vi "Init Runtime.vi"(8 "error in (no error)":errorcluster, 10 "data allocations":T1, 11 "Counter Config in":refnum<class "Counter Config.lvclass">) -> (0 "error out":errorcluster, 2 "Skip":bool, 3 "Counter Config out":refnum<class "Counter Config.lvclass">)   [LabVIEW 2015, in "Counter Config.lvclass"]
uses:
  Counter Config.lvclass
  <vilib>/NI/Tag Bus Module Framework/channel/data tables.ctl
  <vilib>/NI/Tag Bus/dictionary/data dictionary.lvclass
  <vilib>/NI/Tag Bus/dictionary table pair.ctl
  <vilib>/NI/Tag Bus/table/data table.ctl
  Runtime/Counter.lvclass
  <vilib>/NI/Tag Bus/tag/tag descriptor.lvclass/tag descriptor.ctl
  <vilib>/NI/Tag Bus/tag/read tag name.vi
  <vilib>/NI/Tag Bus/tag/read data type.vi
  <vilib>/NI/Tag Bus/dictionary/locate tag.vi
  <vilib>/NI/Tag Bus Module Framework/channel/TBM channel.lvclass
  <vilib>/NI/Tag Bus/table/data table.lvlib
  <vilib>/NI/Tag Bus/tag bus.lvlib
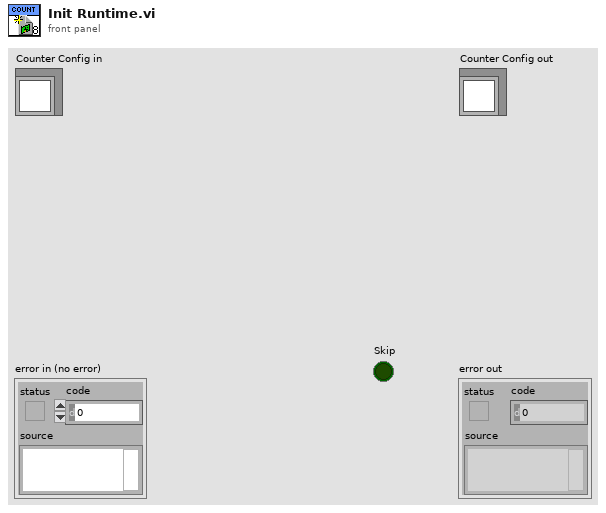
[diagram p1: front panel]
types:
  T1 = typedef "TBM channel.lvclass/data tables.ctl" = cluster{"input data":T2, "processing parameter":T2, "processing result":T2, "output data":T2}
  T2 = typedef "tag bus.lvlib/dictionary table pair.ctl" = cluster{"data dictionary":refnum<class "data dictionary.lvclass">, "data table":T3}
  T3 = typedef "tag bus.lvlib/data table.lvlib/data table.ctl" = cluster{"Double":dbl[], "Single":sgl[], "I64":i64[], "I32":i32[], "I16":i16[], "I8":i8[], "U64":u64[], "U32":u32[], "U16":u16[], "U8":u8[], "Boolean":bool[], "String":string[], "Array of Double":cluster{"DBL Array":dbl[]}[], "Array of Single":cluster{"SGL Array":sgl[]}[], "Array of I64":cluster{"I64 Array":i64[]}[], "Array of I32":cluster{"I32 Array":i32[]}[], "Array of I16":cluster{"I16 Array":i16[]}[], "Array of I8":cluster{"I8 Array":i8[]}[], "Array of U64":cluster{"U64 Array":u64[]}[], "Array of U32":cluster{"U32 Array":u32[]}[], "Array of U16":cluster{"U16 Array":u16[]}[], "Array of U8":cluster{"U8 Array":u8[]}[], "Array of Boolean":cluster{"Boolean Array":bool[]}[], "Array of String":cluster{"String Array":string[]}[]}
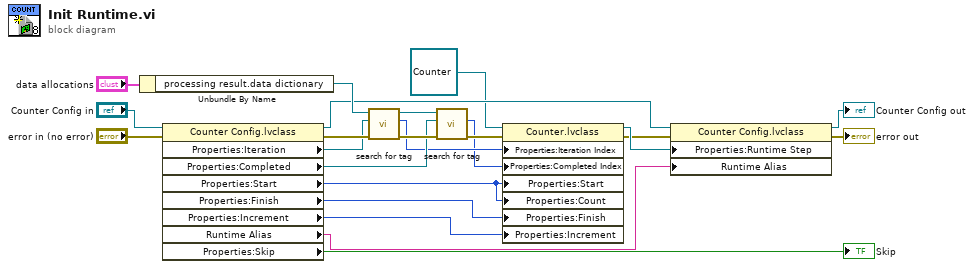
[diagram p0: block diagram]
diagram:
  n1 = Unbundle By Name("data allocations") -> ("processing result.data dictionary"=w19:refnum<class "data dictionary.lvclass">)
  n2 = property class="Counter Config.lvclass"(reference="Counter Config in", error in="error in (no error)") -> (reference out=w17:refnum<class "Counter Config.lvclass">, error out=w10:errorcluster, "Properties:Iteration"=w8:refnum<class "TBM channel.lvclass">, "Properties:Completed"=w7:refnum<class "TBM channel.lvclass">, "Properties:Start"=w4:i32, "Properties:Finish"=w22:i32, "Properties:Increment"=w21:i32, "Runtime Alias"=w2:string, "Properties:Skip"=→"Skip":bool)
  n3 = call <vilib>:"search for tag.vi"("error in"=w10, "system tag"=w8, "data dictionary in"=w19) -> ("error out"=w12:errorcluster, "index"=w6:i32, "data dictionary out"=w18:refnum<class "data dictionary.lvclass">)  [unwired: 6 in]
  n4 = call <vilib>:"search for tag.vi"("error in"=w12, "system tag"=w7, "data dictionary in"=w18) -> ("error out"=w11:errorcluster, "index"=w5:i32)  [unwired: 6 in, 1 out]
  n5 = property class="Counter.lvclass"(reference=refnum<class "Counter.lvclass"> refnum ("Counter.lvclass"), error in=w11, "Properties:Iteration Index"=w6, "Properties:Completed Index"=w5, "Properties:Start"=w4, "Properties:Count"=w4, "Properties:Finish"=w22, "Properties:Increment"=w21) -> (reference out=w16:refnum<class "Counter.lvclass">, error out=w13:errorcluster)
  n6 = property class="Counter Config.lvclass"(reference=w17, error in=w13, "Properties:Runtime Step"=w16, "Runtime Alias"=w2) -> (reference out=→"Counter Config out":refnum<class "Counter Config.lvclass">, error out=→"error out":errorcluster)
